vi "example_drawFlatFrame.vi"() -> ()   [LabVIEW 2023]
uses:
  Ctrls/rectangle.ctl
  BlockDiagram/BlockDiagram.lvclass
  GObject/GObject.lvclass
  TLC_Scripto.lvlib
panel:
  out "unionRect":T1
  out "selectedNumber":i32
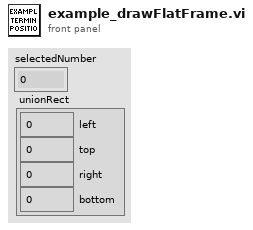
[diagram p1: front panel]
types:
  T1 = typedef "TLC_Scripto.lvlib/rectangle.ctl" = cluster{"left":i32, "top":i32, "right":i32, "bottom":i32}
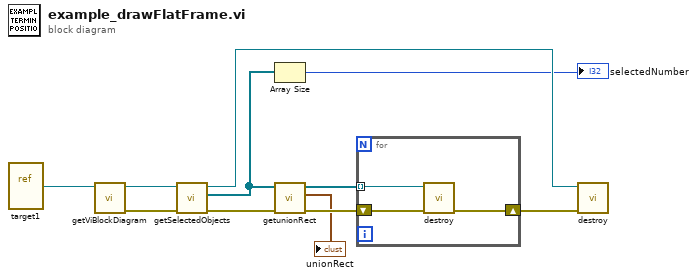
[diagram p0: block diagram]
diagram:
  n1 = vi-ref "target1.vi"() -> (w11:refnum<vi>)
  n2 = call "getViBlockDiagram.vi"("ViRef"=w11) -> ("error out"=w9:errorcluster, "topMostBlockDiagram"=w10:refnum<class "BlockDiagram.lvclass">)  [unwired: 9 in]
  n3 = call "getSelectedObjects.vi"("error in (no error)"=w9, "BlockDiagram in"=w10) -> ("error out"=w3:errorcluster, "selectedGObjects"=w5:refnum<class "GObject.lvclass">[], "BlockDiagram out"=w8:refnum<class "BlockDiagram.lvclass">)  [unwired: 7 in]
  n4 = Array Size(array=w5) -> (size(s)=→"selectedNumber":i32)
  n5 = call "getunionRect.vi"("error in (no error)"=w3, "GObjects"=w5) -> ("error out"=w2:errorcluster, "unionRect"=→"unionRect":T1, "GObjects(dup)"=w4:refnum<class "GObject.lvclass">[])  [unwired: 7 in]
  n6 = for {
    tunnel: w4 -> [w14] mode=indexing
    shift-right: [w13] -> w6
    shift-left: w2 -> [w12]
    n7 = call-dynamic "destroy.vi"("Error In"=w12, "object in"=w14) -> ("Error Out"=w13:errorcluster)  [unwired: 9 in]
  }
  n8 = call-dynamic "destroy.vi"("Error In"=w6, "object in"=w8) -> ()  [unwired: 9 in, 1 out]
